vi "Get Increment (Integer).vi"(8 "error in (no error)":errorcluster, 10 "Feature":string, 11 "Camera in":refnum<class "Camera.lvclass">) -> (0 "error out":errorcluster, 2 "Increment":i64, 3 "Camera":refnum<class "Camera.lvclass">)   [LabVIEW 2020, in "Camera.lvclass"]
uses:
  Camera.lvclass
  Camera.lvclass/Camera.ctl
  bin/gindustrialcam_32-1.dll
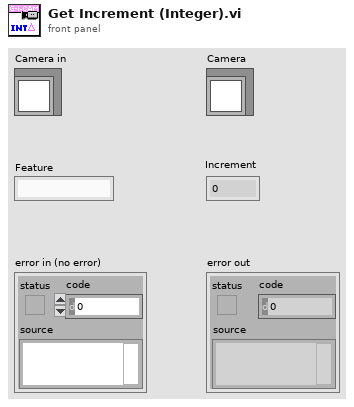
[diagram p1: front panel]
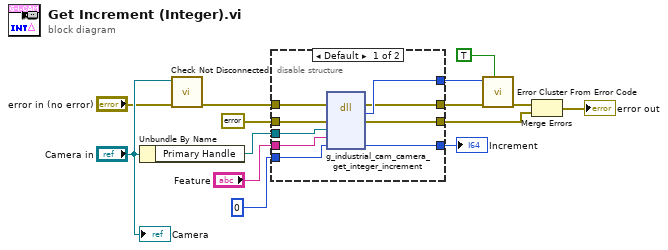
[diagram p0: block diagram]
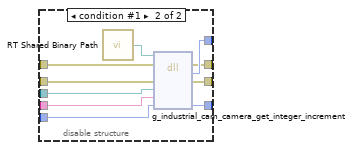
[diagram p2: hidden frame]
diagram:
  n1 = Unbundle By Name("Camera in") -> ("Primary Handle"=w9:refnum<data-value>)
  n2 = call "Check Not Disconnected.vi"("error in (no error)"="error in (no error)", "Camera in"="Camera in") -> ("error out"=w10:errorcluster)  [unwired: 9 in]
  n3 = disable-structure shown="Default" {
    disable-tunnel: [w23 w33] -> w11
    disable-tunnel: w10 -> [w22 w32]
    disable-tunnel: w9 -> [w21 w31]
    disable-tunnel: errorcluster {"status"=FALSE, "code"=0, "source"=""} ("error constant") -> [w20 w30]
    disable-tunnel: [w19 w29] -> w6
    disable-tunnel: [w18 w28] -> w4
    disable-tunnel: [w17 w27] -> w3
    disable-tunnel: i64 0 ("Value In") -> [w16 w26]
    disable-tunnel: "Feature" -> [w15 w25]
    frame condition #0 (active) {
      n4 = dll-call lib="C:/serenial/lib/g-industrial-camera/LabVIEW/g_industrial_cam/bin/gindustrialcam_*-1.*" fn="g_industrial_cam_camera_get_integer_increment"(error in=w22, "err"=w20, "edvr"=w21, "feature"=w15, "increment"=w16) -> (error out=w17:errorcluster, "Mg_Error"=w18:i32, "err"=w19:errorcluster, "increment"=w23:i64)  [unwired: 4 in, 1 out]
    }
    frame condition #1 {
      n5 = call "RT Shared Binary Path.vi"() -> ("Path"=w24:path)
      n6 = dll-call lib="C:/serenial/lib/g-industrial-camera/LabVIEW/g_industrial_cam/bin/gindustrialcam_*-1.*" fn="g_industrial_cam_camera_get_integer_increment"(path in=w24, error in=w32, "err"=w30, "edvr"=w31, "feature"=w25, "increment"=w26) -> (error out=w27:errorcluster, "Mg_Error"=w28:i32, "err"=w29:errorcluster, "increment"=w33:i64)  [unwired: 3 in, 1 out]
    }
  }
  "Increment" <- w11
  n7 = call <vilib>:"Error Cluster From Error Code.vi"("show call chain? (False)"=TRUE, "error in (no error)"=w3, "error code (0)"=w4) -> ("error out"=w5:errorcluster)  [unwired: 6 in]
  n8 = Merge Errors(w5, w6) -> (→"error out":errorcluster)
  "Camera" <- "Camera in"
